vi "Launch Nested Devices.vi"(8 "error in (no error)":errorcluster, 11 "Controller in":refnum<class "Controller.lvclass">) -> (0 "error out":errorcluster, 3 "Controller out":refnum<class "Controller.lvclass">)   [LabVIEW 2014]
uses:
  <vilib>/ActorFramework/Actor/Actor.lvclass
  reusable/DAQ Device/Device/Device.lvclass
  Controller.lvclass
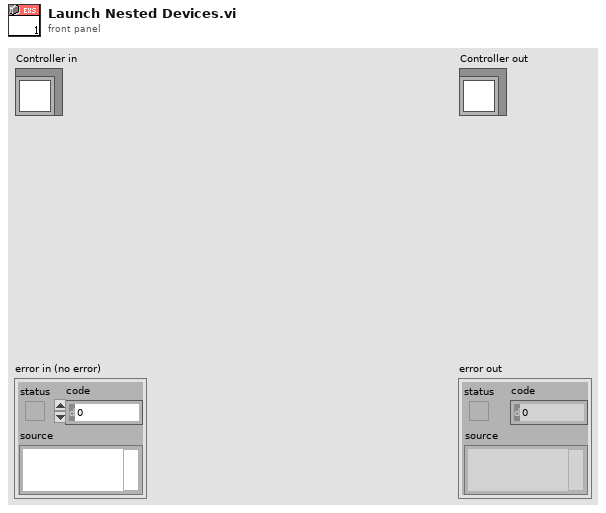
[diagram p1: front panel]
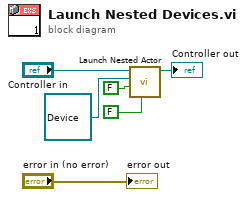
[diagram p0: block diagram]
diagram:
  n1 = call <vilib>:"Launch Nested Actor.vi"("Open Actor Core front panel? (F)"=FALSE, "Auto-stop? (T)"=FALSE, "Nested Actor"=refnum<class "Device.lvclass"> refnum ("DAQ Device.lvlib:Device"), "Caller Actor in"="Controller in") -> ("Caller Actor out"=→"Controller out":refnum<class "Controller.lvclass">)  [unwired: 5 in, 2 out]
  "error out" <- "error in (no error)"
